vi "Perform Work.vi"(4 "Controller name":string, 6 "Last request":bool, 7 "Update period":dbl, 8 "error in (no error)":errorcluster, 9 "Initialize":bool, 11 "Measure Controller in":refnum<class "Monitor Controller.lvclass">) -> (0 "error out":errorcluster, 3 "Measure Controller out":refnum<class "Monitor Controller.lvclass">)   [LabVIEW 2021, in "Monitor Controller.lvclass"]
uses:
  Monitor Controller.lvclass
  C:/GitHub/LabActor/Controllers/Process Controller/Process Controller.lvclass
  Process Controller/Process Controller.lvclass/Process Controller.ctl
  Recorders/Interfaces/Continuous Recorder Messages/Measure Msg/Measure Msg.lvclass/Measure Msg.ctl
  <vilib>/ActorFramework/Message Enqueuer/Message Enqueuer.lvclass/Message Enqueuer.ctl
  Process Controller/Read Active measurements enqueuers.vi
  <vilib>/ActorFramework/Message Enqueuer/Enqueue.vi
  Recorders/Interfaces/Continuous Recorder Messages/Measure Msg/Measure Msg.lvclass
  C:/Program Files/National Instruments/LabVIEW 2021/vi.lib/ActorFramework/Message/Message.lvclass
  <vilib>/ActorFramework/Message Priority Queue/Priority Enqueue.vi
  Process Controller/Process Controller.lvclass
  <vilib>/ActorFramework/Message Enqueuer/Message Enqueuer.lvclass
  Monitor Controller.lvclass/Monitor Controller.ctl
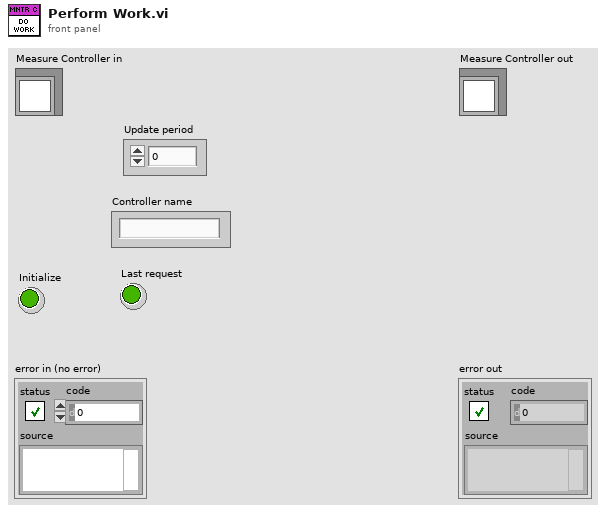
[diagram p1: front panel]
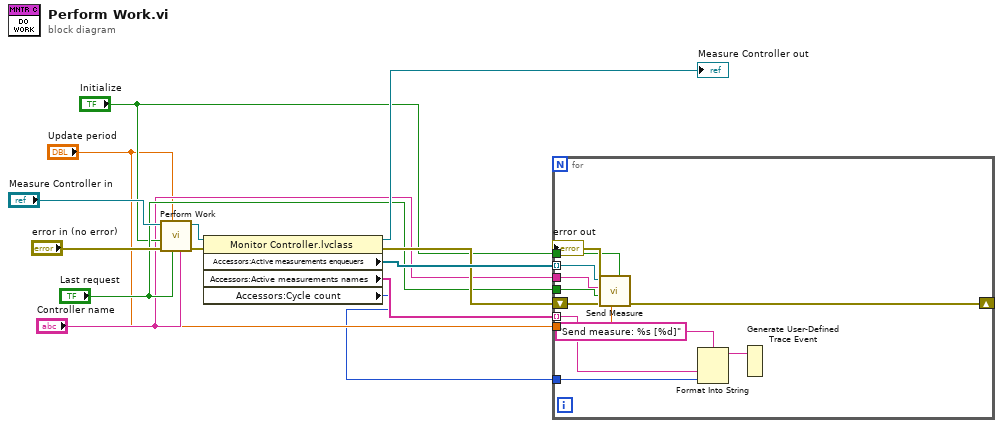
[diagram p0: block diagram]
diagram:
  n1 = call-parent "Perform Work.vi"("Controller name"="Controller name", "Last request"="Last request", "Update period"="Update period", "error in (no error)"="error in (no error)", "Initialize"="Initialize", "Measure Controller in"="Measure Controller in") -> ("error out"=w8:errorcluster, "Measure Controller out"=w10:refnum<class "Monitor Controller.lvclass">)  [unwired: 4 in]
  n2 = property class="Monitor Controller.lvclass"(reference=w10, error in=w8) -> (reference out=→"Measure Controller out":refnum<class "Monitor Controller.lvclass">, error out=w11:errorcluster, "Accessors:Active measurements enqueuers"=w12:refnum<class "Message Enqueuer.lvclass">[], "Accessors:Active measurements names"=w2:string[], "Accessors:Cycle count"=w1:i32)
  n3 = for {
    tunnel: w12 -> [w25] mode=indexing
    tunnel: "Controller name" -> [w24]
    shift-right: [w20] -> w7
    shift-left: w11 -> [w23]
    tunnel: "Update period" -> [w22]
    tunnel: "Last request" -> [w21]
    tunnel: "Initialize" -> [w19]
    tunnel: w2 -> [w16] mode=indexing
    tunnel: w1 -> [w15]
    n4 = call "Send Measure.vi"("Init work"=w19, "Update period"=w22, "error in (no error)"=w23, "Last request"=w21, "Requester"=w24, "Message Enqueuer"=w25) -> ("error out"=w20:errorcluster)  [unwired: 4 in, 1 out]
    n5 = Format Into String(format string="Send measure: %s [%d]", w16, w15) -> (resulting string=w17:string)  [unwired: 2 in, 1 out]
    n6 = Generate User-Defined Trace Event(2:w17) -> ()  [unwired: 1 in]
  }
  "error out" <- w7
